vi "GenericBlastPulseWithTransducer.vi"() -> ()   [LabVIEW 2015]
doc: "The UDP protocol differs from TCP in that there is no error-checking with the packets of information that are sent, and thus no guarantee whatsoever that an intended recipient will actually receive a given piece of data.\n\nUDP does offer the ability to \"broadcast\" data across a network--simply specify an IP Address of all ones (255.255.255.255) to attempt to broadcast information network-wide. Keep in mind that routers and other network hardware will generally refuse to forward the broadcast beyond certain points, so the extent of the broadcast will in practice be limited."
uses:
  <vilib>/Utility/file.llb/Write To Spreadsheet File (DBL).vi
panel:
  out "Most Recent Blast Profile":dbl[](graph)
  out "Honeywell Pressure Transducer":dynamicdata(graph)
  out "Blast Max Value":dbl
  in  "file path":path=path "C:/Users/bernara2/test.txt"
  in  "Blast":bool
  in  "Sampling Rate":dbl=2000.0 caption="Sampling Rate (hz)"
  in  "stop":bool
  in  "Solenoid Close time":dbl=0.009 caption="(Default 0.009 Seconds)"
  in  "Solenoid Idle Time":dbl=0.008 caption="(Default 0.008 Seconds)"
  in  "Solenoid Open Time":dbl=0.004 caption="(Default 0.004 Seconds)"
  in  "Number of Blasts":dbl=1.0
  in  "Blast Interval (Seconds)":dbl=1.0
  # "Most Recent Blast Waveform"
  # "Instructions:\n\n1. Make sure the BeagleBone Blue board is connected to the paintball gun \nand is powered on.\n\n2. Connect wifi to the BeagleBone-F61D network (password: BeagleBone)\n \n3. Start the VI with the RUN arrow in the top left of the screen\n\n4. Enter blast characteristics and sampling rate\n\n5. Enter a file name in \"file path\" to write data to\n\n6. Click \"Blast\" to start the blast pulse and collect data  \n\n7. Rename \"file path\" to a new file (else data will be overwritten)\n\n8. When finished, click \"STOP RUNNING\"."
  # "Pressure Data (Continuous)"
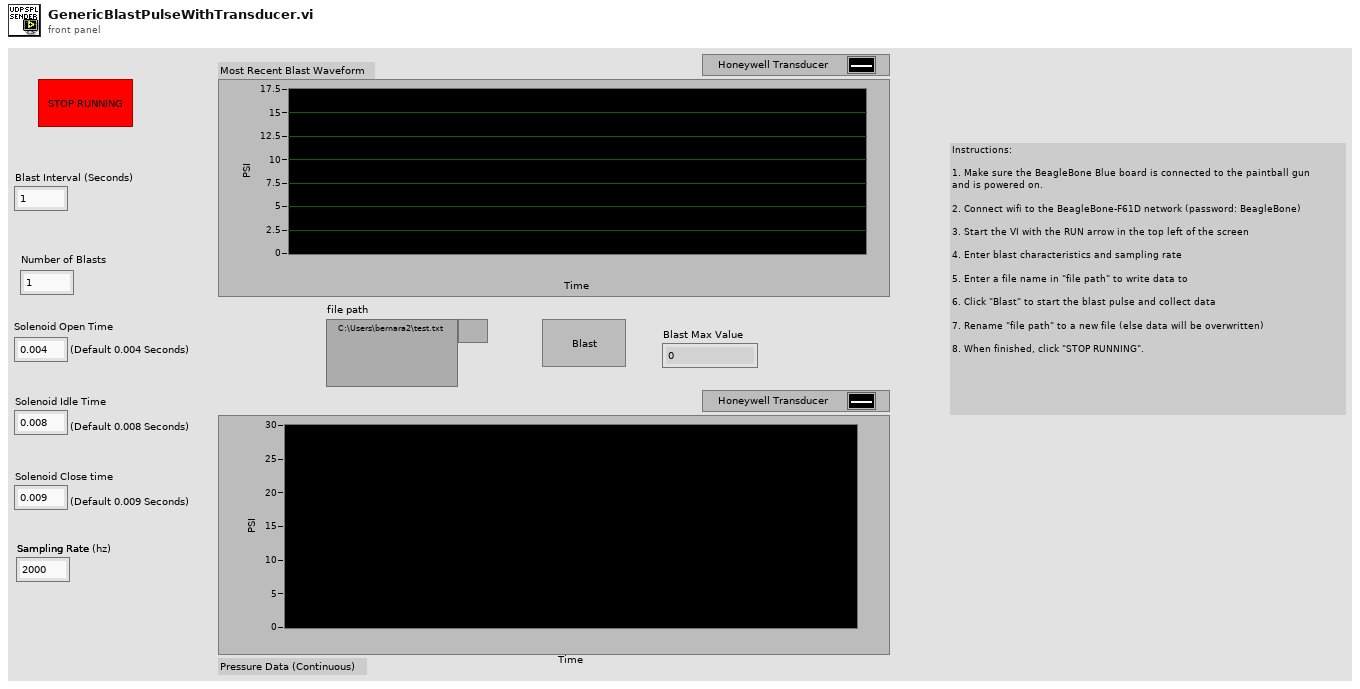
[diagram p1: front panel]
types:
  T1 = enum8{"Enabled", "Disabled", "Disabled and Grayed Out"}
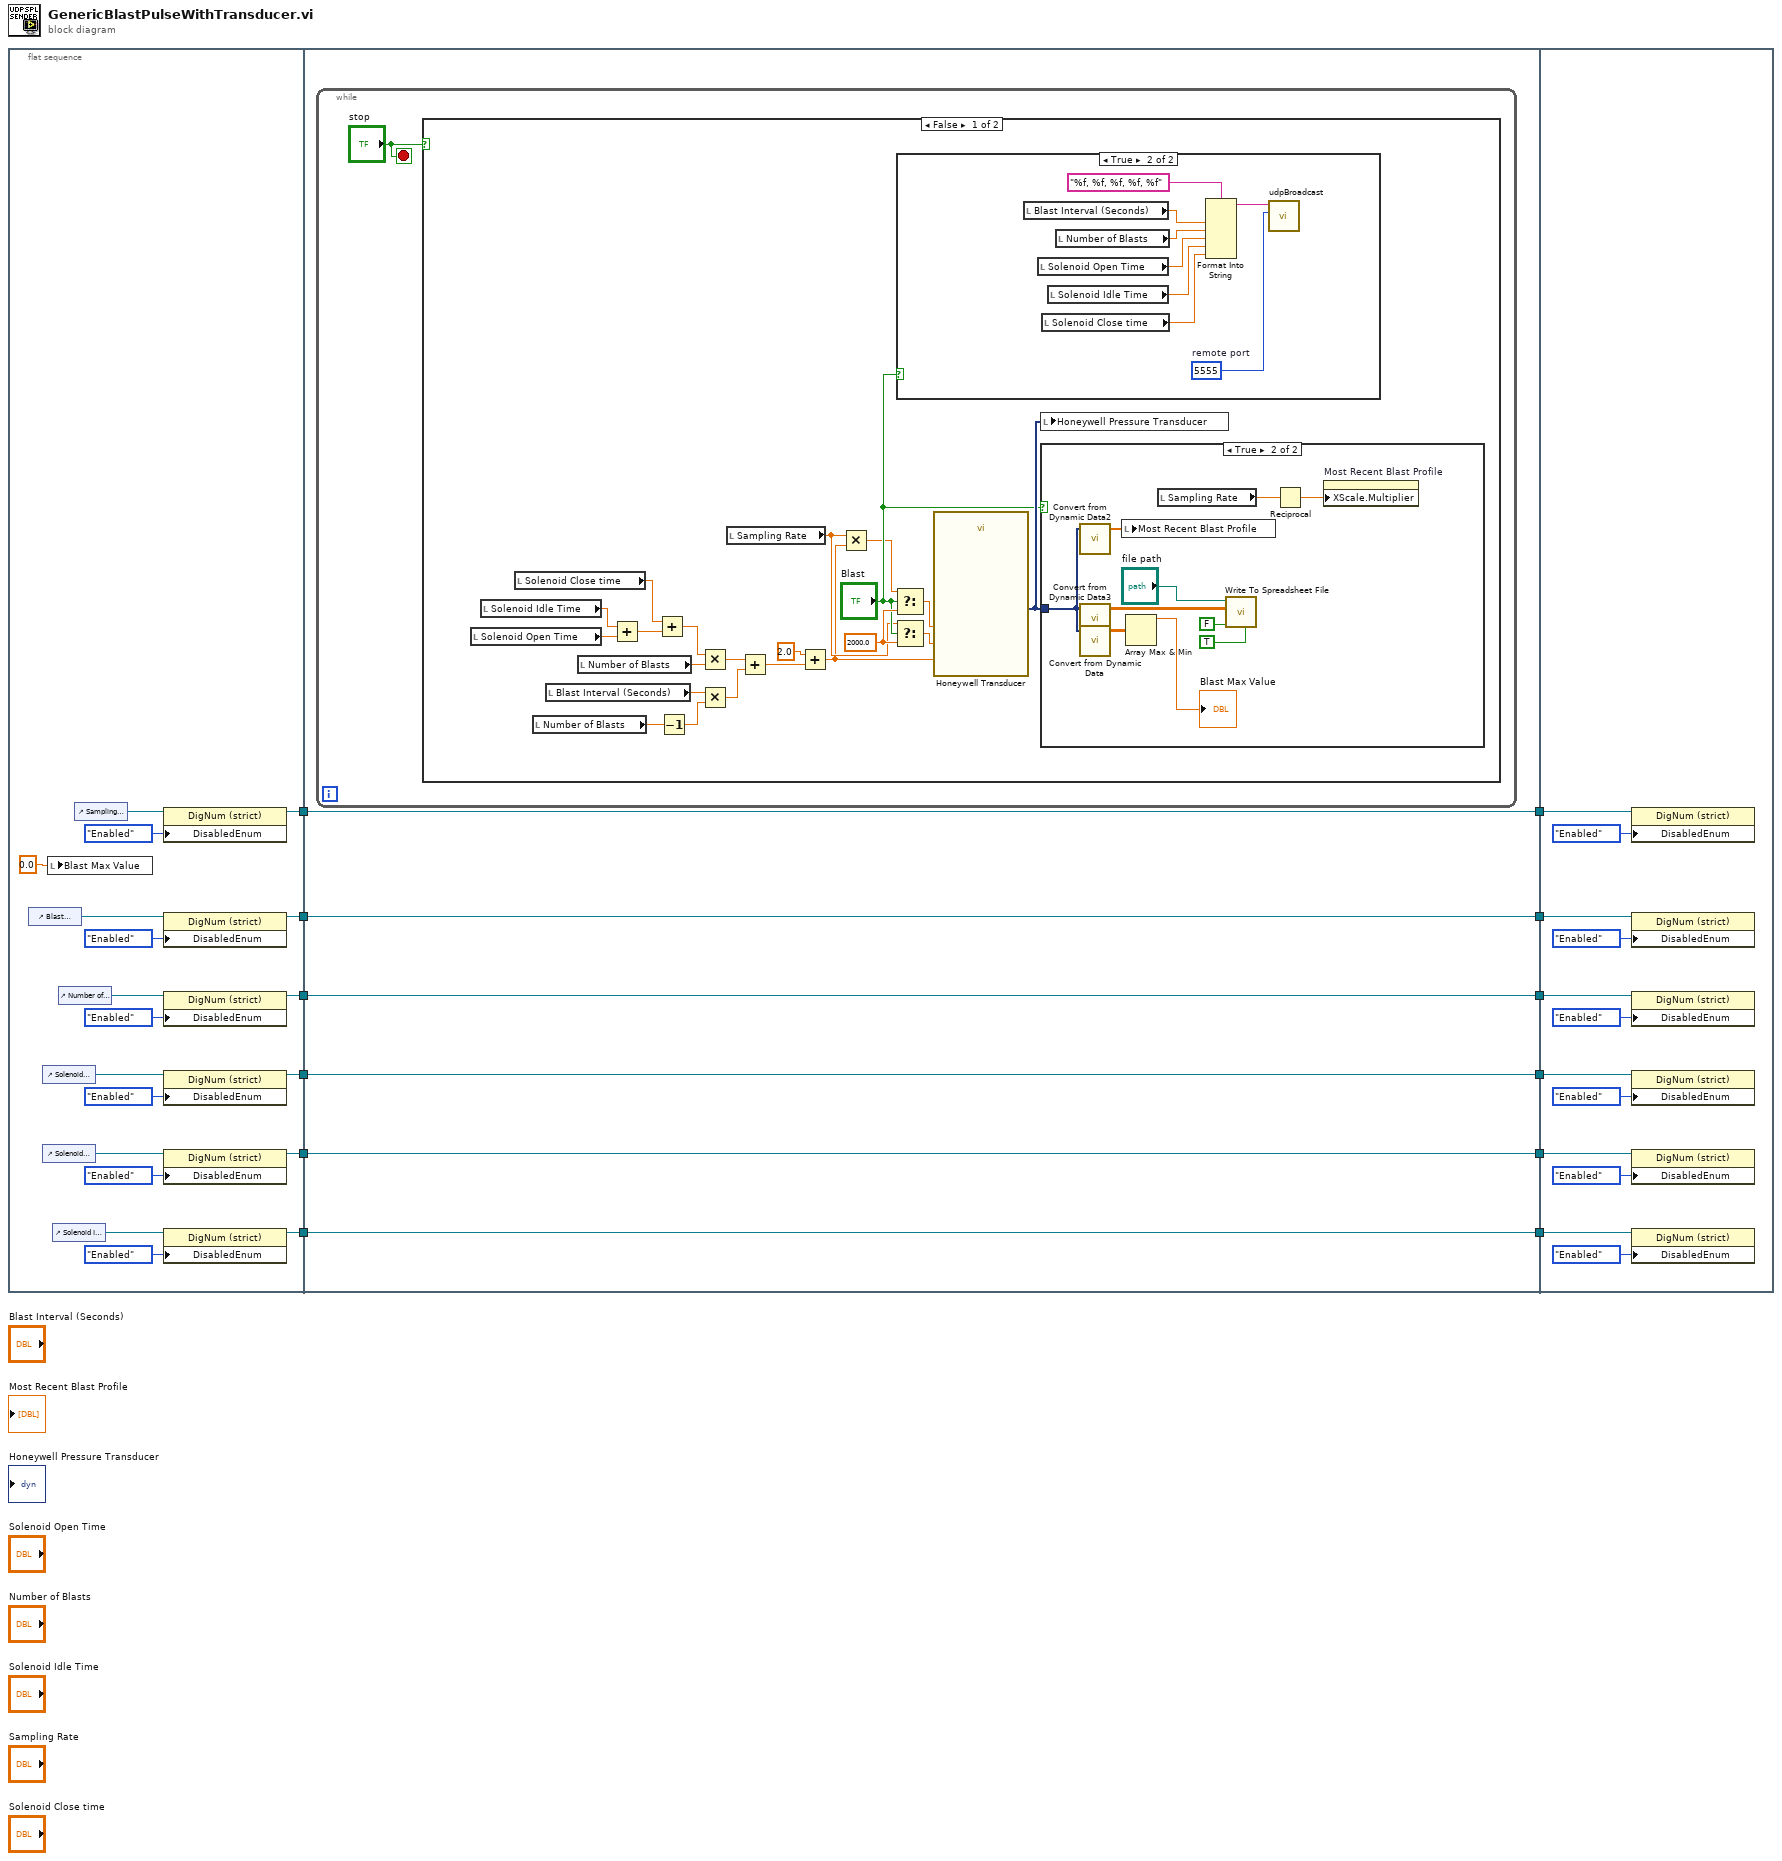
[diagram p0: block diagram]
diagram:
  n1 = flat-sequence {
    tunnel: [w19] -> w11
    tunnel: [w18] -> w9
    tunnel: [w17] -> w7
    tunnel: [w16] -> w5
    tunnel: [w15] -> w3
    tunnel: [w14] -> w1
    tunnel: [w37] -> w12
    tunnel: w11 -> [w37]
    tunnel: [w36] -> w10
    tunnel: w9 -> [w36]
    tunnel: [w35] -> w8
    tunnel: w7 -> [w35]
    tunnel: [w34] -> w6
    tunnel: w5 -> [w34]
    tunnel: [w33] -> w4
    tunnel: w3 -> [w33]
    tunnel: [w32] -> w2
    tunnel: w1 -> [w32]
    tunnel: w12 -> [w83]
    tunnel: w10 -> [w82]
    tunnel: w8 -> [w81]
    tunnel: w6 -> [w80]
    tunnel: w4 -> [w79]
    tunnel: w2 -> [w78]
    frame #0 {
      n2 = control-ref of="Blast Interval (Seconds)"() -> (w31:refnum<vi>)
      n3 = control-ref of="Solenoid Open Time"() -> (w27:refnum<vi>)
      n4 = control-ref of="Solenoid Close time"() -> (w23:refnum<vi>)
      n5 = local write "Blast Max Value"(0.0 ("Most Recent Max Value")) -> ()
      n6 = control-ref of="Solenoid Idle Time"() -> (w24:refnum<vi>)
      n7 = control-ref of="Number of Blasts"() -> (w28:refnum<vi>)
      n8 = control-ref of="Sampling Rate"() -> (w20:refnum<vi>)
      n9 = property class="DigNum (strict)"(reference=w20, "DisabledEnum"=T1."Enabled" ("Disabled")) -> (reference out=w14:refnum<vi>)  [unwired: 1 in, 1 out]
      n10 = property class="DigNum (strict)"(reference=w31, "DisabledEnum"=T1."Enabled" ("Disabled")) -> (reference out=w19:refnum<vi>)  [unwired: 1 in, 1 out]
      n11 = property class="DigNum (strict)"(reference=w28, "DisabledEnum"=T1."Enabled" ("Disabled")) -> (reference out=w18:refnum<vi>)  [unwired: 1 in, 1 out]
      n12 = property class="DigNum (strict)"(reference=w27, "DisabledEnum"=T1."Enabled" ("Disabled")) -> (reference out=w17:refnum<vi>)  [unwired: 1 in, 1 out]
      n13 = property class="DigNum (strict)"(reference=w23, "DisabledEnum"=T1."Enabled" ("Disabled")) -> (reference out=w15:refnum<vi>)  [unwired: 1 in, 1 out]
      n14 = property class="DigNum (strict)"(reference=w24, "DisabledEnum"=T1."Enabled" ("Disabled")) -> (reference out=w16:refnum<vi>)  [unwired: 1 in, 1 out]
    }
    frame #1 {
      n15 = while {
        stop <- "stop" stop-if-true
        n16 = case shown="False" "stop" {
          frame False {
            w51 = 2000.0 ("f")
            n17 = local read "Solenoid Open Time"() -> (w54:dbl)
            n18 = local read "Solenoid Idle Time"() -> (w53:dbl)
            n19 = local read "Solenoid Close time"() -> (w52:dbl)
            n20 = local read "Number of Blasts"() -> (w40:dbl)
            n21 = local read "Blast Interval (Seconds)"() -> (w56:dbl)
            n22 = local read "Number of Blasts"() -> (w57:dbl)
            n23 = Add(x=w53, y=w54) -> (x+y=w58:dbl)
            n24 = Add(x=w52, y=w58) -> (x+y=w59:dbl)
            n25 = Decrement(x=w40) -> (x-1=w39:dbl)
            n26 = Multiply(x=w59, y=w57) -> (x*y=w55:dbl)
            n27 = Multiply(x=w56, y=w39) -> (x*y=w46:dbl)
            n28 = local read "Sampling Rate"() -> (w43:dbl)
            n29 = Add(x=w55, y=w46) -> (x+y=w44:dbl)
            n30 = Add(x=2.0 ("y"), y=w44) -> (x+y=w41:dbl)
            n31 = Multiply(x=w43, y=w41) -> (x*y=w42:dbl)
            n32 = Select(t=w42, s="Blast", f=w51) -> (s? t:f=w50:dbl)
            n33 = Select(t=w43, s="Blast", f=w51) -> (s? t:f=w49:dbl)
            n34 = case shown="True" "Blast" {
              frame False {
              }
              frame True {
                w77 = u16 5555  # remote port
                n35 = local read "Blast Interval (Seconds)"() -> (w74:dbl)
                n36 = local read "Solenoid Open Time"() -> (w72:dbl)
                n37 = local read "Solenoid Close time"() -> (w70:dbl)
                n38 = local read "Solenoid Idle Time"() -> (w71:dbl)
                n39 = local read "Number of Blasts"() -> (w73:dbl)
                n40 = Format Into String(format string="%f, %f, %f, %f, %f", w74, w73, w72, w71, w70) -> (resulting string=w75:string)  [unwired: 2 in, 1 out]
                n41 = call "udpBroadcast.vi"("remote port"=w77, "data in"=w75) -> ()  [unwired: 10 in]
              }
            }
            n42 = call "Honeywell Transducer"("rate"=w49, "number of samples"=w50, "timeout (s)"=w41) -> ("data"=w48:dynamicdata)  [unwired: 13 in, 3 out]
            n43 = local write "Honeywell Pressure Transducer"(w48) -> ()
            n44 = case shown="True" "Blast" {
              tunnel: w48 -> [_ w60]
              frame False {
              }
              frame True {
                n45 = call "Convert from Dynamic Data2"("Dynamic Data Type"=w60) -> ("Array"=w63:dbl[])  [unwired: 3 in]
                n46 = call "Convert from Dynamic Data3"("Dynamic Data Type"=w60) -> ("Array"=w61:dbl[][])  [unwired: 3 in]
                n47 = call "Convert from Dynamic Data"("Dynamic Data Type"=w60) -> ("Array"=w64:dbl[][])  [unwired: 3 in]
                n48 = local write "Most Recent Blast Profile"(w63) -> ()
                n49 = Array Max & Min(array=w64) -> (max value=→"Blast Max Value":dbl)  [unwired: 3 out]
                n50 = local read "Sampling Rate"() -> (w65:dbl)
                n51 = call-poly <vilib>:"Write To Spreadsheet File.vi"("transpose? (no:F)"=TRUE, "append to file? (new file:F)"=FALSE, "2D data"=w61, "file path (dialog if empty)"="file path") -> ()  [unwired: 4 in, 1 out]
                n52 = Reciprocal(x=w65) -> (1/x=w62:dbl)
                n53 = property on="Most Recent Blast Profile" class="WFGraph (strict)"("XScale.Multiplier"=w62) -> ()  [unwired: 2 in, 2 out]
              }
            }
          }
          frame True {
          }
        }
      }
    }
    frame #2 {
      n54 = property class="DigNum (strict)"(reference=w78, "DisabledEnum"=T1."Enabled" ("Disabled")) -> ()  [unwired: 1 in, 2 out]
      n55 = property class="DigNum (strict)"(reference=w83, "DisabledEnum"=T1."Enabled" ("Disabled")) -> ()  [unwired: 1 in, 2 out]
      n56 = property class="DigNum (strict)"(reference=w82, "DisabledEnum"=T1."Enabled" ("Disabled")) -> ()  [unwired: 1 in, 2 out]
      n57 = property class="DigNum (strict)"(reference=w81, "DisabledEnum"=T1."Enabled" ("Disabled")) -> ()  [unwired: 1 in, 2 out]
      n58 = property class="DigNum (strict)"(reference=w79, "DisabledEnum"=T1."Enabled" ("Disabled")) -> ()  [unwired: 1 in, 2 out]
      n59 = property class="DigNum (strict)"(reference=w80, "DisabledEnum"=T1."Enabled" ("Disabled")) -> ()  [unwired: 1 in, 2 out]
    }
  }
